vi "Helmholtz2D_FEM_Check Grid.vi"(8 "Yi In":dbl[](array[numeric]), 9 "Xi In":dbl[](array[numeric]), 10 "Y":dbl[](array[numeric]), 11 "X":dbl[](array[numeric])) -> (2 "Yi Out":dbl[](array[numeric]), 3 "Xi Out":dbl[](array[numeric]))   [LabVIEW 2020, in "NI_PDE.lvlib"]
uses:
  <vilib>/gmath/NI_PDE.lvlib
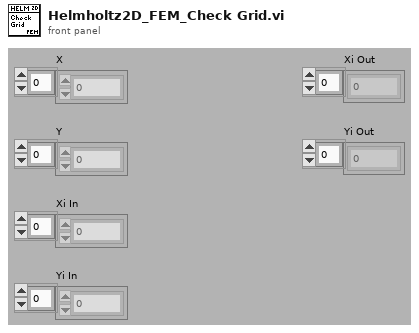
[diagram p1: front panel]
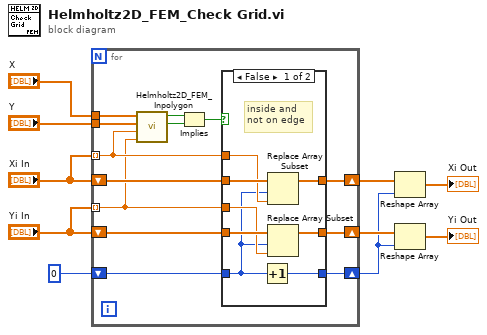
[diagram p0: block diagram]
diagram:
  n1 = for {
    tunnel: "X" -> [w23]
    tunnel: "Y" -> [w22]
    tunnel: "Xi In" -> [w21] mode=indexing
    tunnel: "Yi In" -> [w19] mode=indexing
    shift-right: [w16] -> w4
    shift-left: "Yi In" -> [w18]
    shift-right: [w17] -> w5
    shift-left: "Xi In" -> [w20]
    shift-right: [w14] -> w1
    shift-left: 0 -> [w15]
    n2 = call <vilib>:"Helmholtz2D_FEM_Inpolygon.vi"("yi"=w19, "xi"=w21, "Y"=w22, "X"=w23) -> ("on edge?"=w13:bool, "inside?"=w12:bool)  [unwired: 6 out]
    n3 = Implies(1:w13, 2:w12) -> (0:w11:bool)
    n4 = case shown="False" w11 {
      tunnel: w21 -> [w30 _]
      tunnel: w20 -> [w31 w34]
      tunnel: w19 -> [w28 _]
      tunnel: w18 -> [w29 w33]
      tunnel: [w27 w34] -> w17
      tunnel: [w26 w33] -> w16
      tunnel: w15 -> [w25 w32]
      tunnel: [w24 w32] -> w14
      frame False {
        # "inside and\nnot on edge"
        n5 = Increment(x=w25) -> (x+1=w24:i32)
        n6 = Replace Array Subset(array=w31, new element=w30, index=w25) -> (w27:dbl[])
        n7 = Replace Array Subset(array=w29, new element=w28, index=w25) -> (w26:dbl[])
      }
      frame True {
      }
    }
  }
  n8 = Reshape Array(w5, w1) -> (→"Xi Out":dbl[])
  n9 = Reshape Array(w4, w1) -> (→"Yi Out":dbl[])
